vi "Large integer U8 array - remove ending 0.vi"(5 "Large number - U8":T1) -> (1 "MSD zeros removed":T1)   [LabVIEW 2012]
doc: "Removes any zero elements at end of U8 array in a large numbers (U8 array format). If all elements are zero it returns an array of 1 element = 0."
uses:
  User Access Type defs/Large number - U8 array.ctl
panel:
  # "index 0 = LSD"
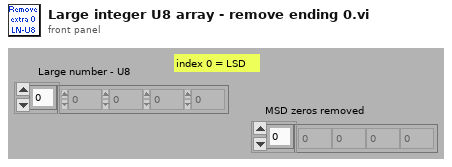
[diagram p1: front panel]
types:
  T1 = typedef "Large number - U8 array.ctl" = u8[]
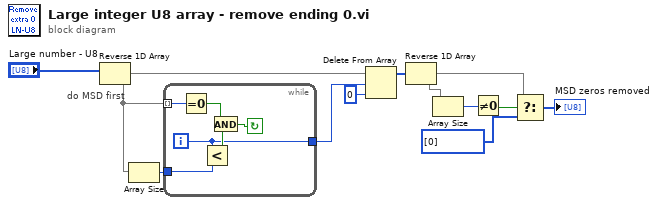
[diagram p0: block diagram]
diagram:
  # "do MSD first"
  n1 = Reverse 1D Array(array="Large number - U8") -> (reversed array=w10:T1)
  n2 = Array Size(array=w10) -> (size(s)=w9:i32)
  n3 = while {
    tunnel: w10 -> [w17] mode=indexing
    tunnel: w9 -> [w15]
    tunnel: [w12] -> w6
    i -> [w12]
    stop <- w16 continue-if-true
    n4 = Equal To 0?(x=w17) -> (x = 0?=w13:bool)
    n5 = Less?(x=w12, y=w15) -> (x < y?=w14:bool)
    n6 = And(x=w13, y=w14) -> (x .and. y?=w16:bool)
  }
  n7 = Delete From Array(array=w10, length=w6, index=0) -> (array with subset deleted=w7:T1)  [unwired: 1 out]
  n8 = Reverse 1D Array(array=w7) -> (reversed array=w5:T1)
  n9 = Array Size(array=w5) -> (size(s)=w4:i32)
  n10 = Not Equal To 0?(x=w4) -> (x != 0?=w3:bool)
  n11 = Select(t=w5, s=w3, f=u8[] [0]) -> (s? t:f=→"MSD zeros removed":T1)
